vi "Create_directory_path.vi"(2 "error in (no error)":errorcluster, 3 "Dialog Box":bool=TRUE, 4 "Path name":path) -> (0 "error out":errorcluster, 1 "Path name Out":path)   [LabVIEW 2021]
panel:
  out "length":i32
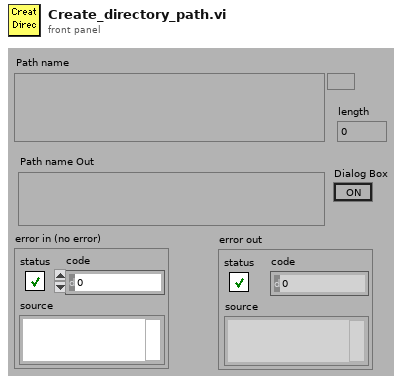
[diagram p1: front panel]
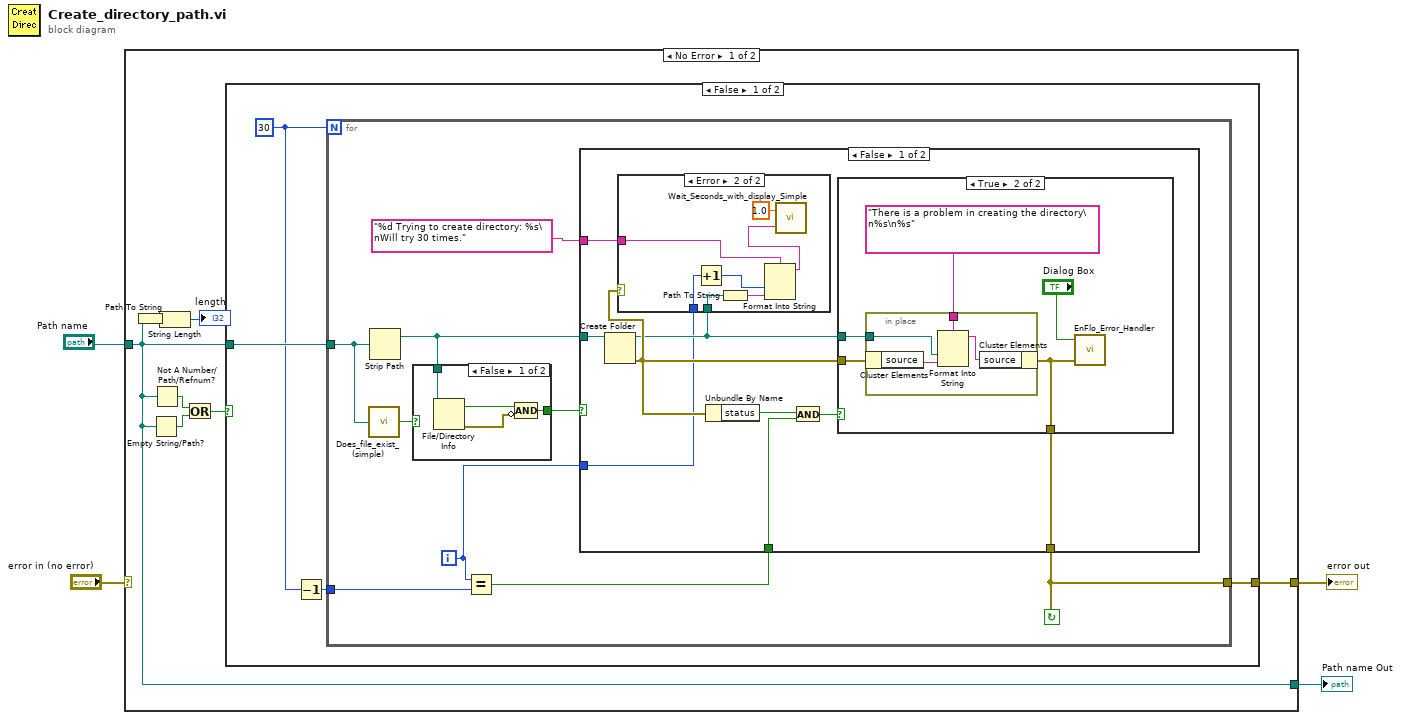
[diagram p0: block diagram]
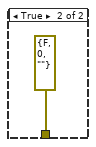
[diagram p4: hidden frame]
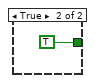
[diagram p5: hidden frame]
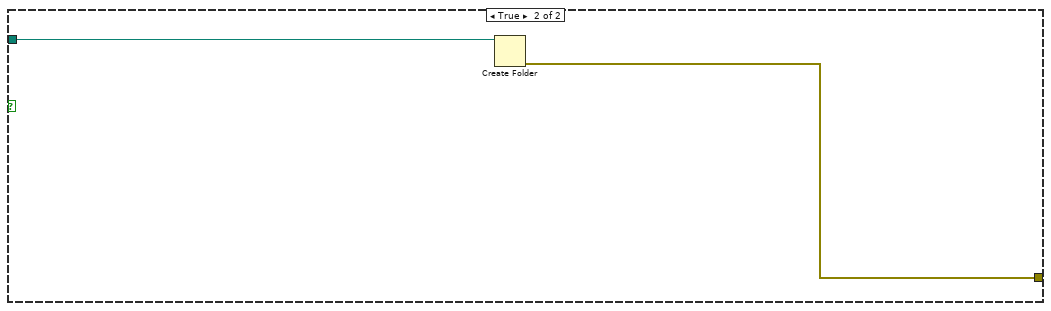
[diagram p6: hidden frame]
diagram:
  n1 = case shown="No Error" "error in (no error)" {
    selector: "error in (no error)" -> [_ w59]
    tunnel: [w11 w59] -> w4
    tunnel: "Path name" -> [w7 w60]
    tunnel: [w7 w60] -> w1
    frame No Error {
      n2 = Path To String(path=w7) -> (string=w5:string)
      n3 = Empty String/Path?(string/path=w7) -> (empty?=w10:bool)
      n4 = Not A Number/Path/Refnum?(number/path/refnum=w7) -> (NaN/Path/Refnum?=w9:bool)
      n5 = String Length(string=w5) -> (length=→"length":i32)
      n6 = Or(x=w9, y=w10) -> (x .or. y?=w8:bool)
      n7 = case shown="False" w8 {
        tunnel: [w15 w57] -> w11
        tunnel: w7 -> [w13 w58]
        frame False {
          w12 = 30
          n8 = Decrement(x=w12) -> (x-1=w14:i32)
          n9 = for {
            N: w12 -> [_]
            tunnel: [w18] -> w15
            tunnel: w13 -> [w21]
            tunnel: w14 -> [w20]
            i -> [w17]
            stop <- w18 continue-if-true
            n10 = call "Does_file_exist_(simple).vi"("Pathname"=w21) -> ("exists?"=w22:bool)
            n11 = Strip Path(path=w21) -> (stripped path=w23:path)  [unwired: 1 out]
            n12 = case shown="False" w22 {
              tunnel: [w55 TRUE] -> w24
              tunnel: w23 -> [w53 _]
              frame False {
                n13 = File/Directory Info(path=w53) -> (directory=w54:bool, error out=w52:errorcluster)  [unwired: 1 in, 5 out]
                n14 = Compound Arithmetic op=AND(w54, invert w52) -> (w55:bool)
              }
              frame True {
              }
            }
            n15 = Equal?(x=w17, y=w20) -> (x = y?=w19:bool)
            n16 = case shown="False" w24 {
              tunnel: w23 -> [w29 _]
              tunnel: [w33 errorcluster {"status"=FALSE, "code"=0, "source"=""} ("error in (no error)")] -> w18
              tunnel: w19 -> [w31 _]
              tunnel: w17 -> [w26 _]
              tunnel: "%d Trying to create directory: %s\nWill try 30 times." ("format string") -> [w25 _]
              frame False {
                n17 = Create Folder(path (use dialog)=w29) -> (created path=w27:path, error out=w28:errorcluster)  [unwired: 2 in, 1 out]
                n18 = case shown="Error" w28 {
                  tunnel: w27 -> [_ w39]
                  tunnel: w26 -> [_ w37]
                  tunnel: w25 -> [_ w34]
                  frame No Error {
                  }
                  frame Error {
                    n19 = Increment(x=w37) -> (x+1=w36:i32)
                    n20 = Path To String(path=w39) -> (string=w35:string)
                    n21 = Format Into String(format string=w34, w36, w35) -> (resulting string=w38:string)  [unwired: 2 in, 1 out]
                    n22 = call "Wait_Seconds_with_display_Simple.vi"("Message"=w38, "Seconds to wait"=1.0) -> ()  [unwired: 1 in, 1 out]
                  }
                }
                n23 = Unbundle By Name(w28) -> ("status"=w32:bool)
                n24 = And(x=w32, y=w31) -> (x .and. y?=w30:bool)
                n25 = case shown="True" w30 {
                  tunnel: w27 -> [_ w43]
                  tunnel: [w41 w42] -> w33
                  tunnel: w28 -> [w41 w45]
                  frame False {
                  }
                  frame True {
                    n26 = in-place {
                      in-place-border: "There is a problem in creating the directory\n%s\n%s" ("format string") -> [w50]
                      in-place-border: w43 -> [w49]
                      n27 = in-place-cluster #1(w45) -> ("source"=w48:string)
                      n28 = Format Into String(format string=w50, w49, w48) -> (resulting string=w47:string)  [unwired: 2 in, 1 out]
                      n29 = in-place-cluster #1("source"=w47) -> (w42:errorcluster)
                    }
                    n30 = call "EnFlo_Error_Handler.vi"("error in (no error)"=w42, "Dialog Box (F)"="Dialog Box") -> ()  [unwired: 1 in, 3 out]
                  }
                }
              }
              frame True {
              }
            }
          }
        }
        frame True {
          n31 = Create Folder(path (use dialog)=w58) -> (error out=w57:errorcluster)  [unwired: 2 in, 2 out]
        }
      }
    }
    frame Error {
    }
  }
  "error out" <- w4
  "Path name Out" <- w1
